vi "Init Stim Param Display.vi"(4 "Left Train length":i64[](array[numeric]), 5 "Left Stim Params in":T1) -> (2 "Left Stim Params out":T3)   [LabVIEW 2019]
uses:
  Controls/Type Defs/Stim Parameters.ctl
  Controls/Stim off-half-ful.ctl
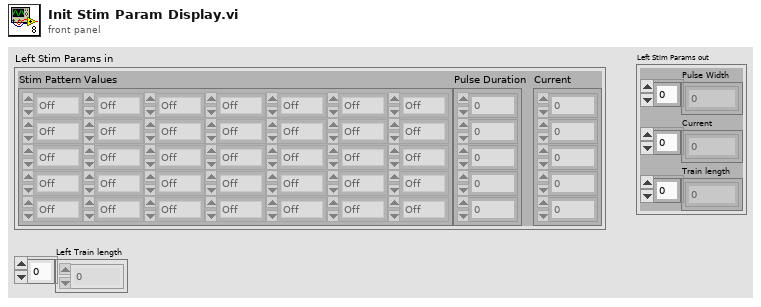
[diagram p1: front panel]
types:
  T1 = typedef "Stim Parameters.ctl" = cluster{"Stim Pattern Values":T2[][], "Pulse Duration":i64[], "Current":i64[]}
  T2 = typedef "Stim off-half-ful.ctl" = enum16{"Off", "Half", "Full"}
  T3 = cluster{"Pulse Width":i64[], "Current":i64[], "Train length":i64[]}
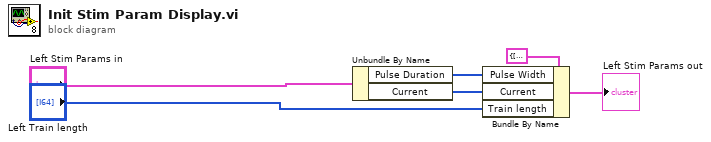
[diagram p0: block diagram]
diagram:
  n1 = Unbundle By Name("Left Stim Params in") -> ("Pulse Duration"=w4:i64[], "Current"=w5:i64[])
  n2 = Bundle By Name(cluster=T3 {"Pulse Width"=[20, 200, 200, 200, 200], "Current"=[20, 20, 20, 20, 20], "Train length"=[200, 200, 200, 200, 200, 114, 214, 314, 414, 514]} ("Left Stim Params"), "Pulse Width"=w4, "Current"=w5, "Train length"="Left Train length") -> (→"Left Stim Params out":T3)
